vi "Sub_Truncate_2D.vi"(10 "samples":i32, 11 "?":dbl[][](array[numeric])) -> (3 "array":dbl[][](array[numeric]))   [LabVIEW 2021]
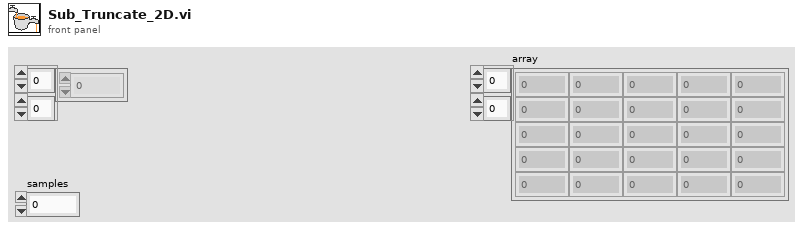
[diagram p1: front panel]
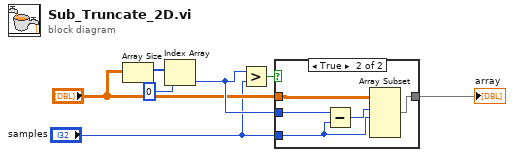
[diagram p0: block diagram]
diagram:
  n1 = Array Size(array="?") -> (size(s)=w5:i32[])
  n2 = Index Array(array=w5, index=0) -> (element=w3:i32)
  n3 = Greater?(x=w3, y="samples") -> (0:w7:bool)
  n4 = case shown="True" w7 {
    tunnel: "samples" -> [_ w9]
    tunnel: "?" -> [w8 w13]
    tunnel: [w8 w12] -> w6
    tunnel: w3 -> [_ w11]
    frame False {
    }
    frame True {
      n5 = Subtract(x=w11, y=w9) -> (x-y=w10:i32)
      n6 = Array Subset(array=w13, index (row)=w10, length (row)=w9) -> (w12:dbl[][])  [unwired: 2 in]
    }
  }
  "array" <- w6
